vi "Setra Close.vi"(8 "Error In":errorcluster, 11 "VISA Refnum in":refnum<visa-resource-name>) -> (0 "Error Out":errorcluster)   [LabVIEW 2019]
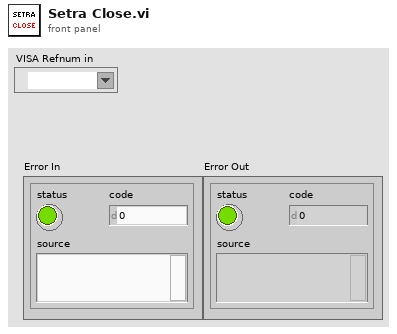
[diagram p1: front panel]
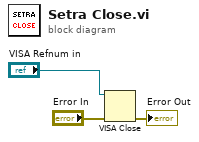
[diagram p0: block diagram]
diagram:
  n1 = VISA Close(VISA resource name="VISA Refnum in", error in (no error)="Error In") -> (error out=→"Error Out":errorcluster)
